vi "Create From Elements.vi"(7 "Mutable (F)":bool, 8 "error in (no error)":errorcluster, 10 "Elements":T1[](array[typedef])) -> (0 "error out":errorcluster, 3 "Config Manager out":refnum<class "Config Manager.lvclass">)   [LabVIEW 2023, in "CDM-Config.lvlib" / "Config Manager.lvclass"]
uses:
  Config Manager.lvclass
  Config Element.ctl
  Meta Data.ctl
  Value Type.ctl
  Config Element/Element Data.ctl
  Node Info.ctl
  Config Manager.lvclass/Config Manager.ctl
  CDM-Config.lvlib
  Config Element/Config Element.lvclass
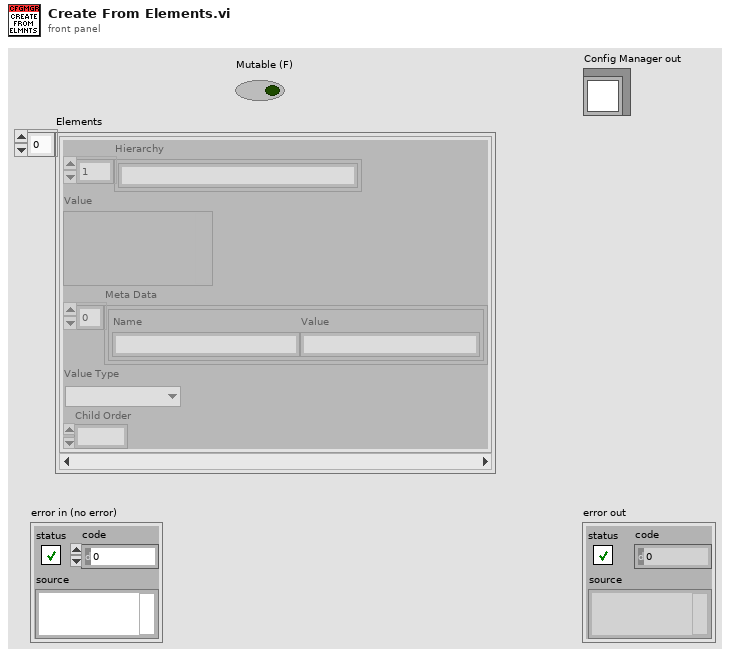
[diagram p1: front panel]
types:
  T1 = typedef "CDM-Config.lvlib/Config Element.ctl" = cluster{"Hierarchy":string[], "Value":variant, "Meta Data":T2[], "Value Type":T3, "Child Order":i32}
  T2 = typedef "CDM-Config.lvlib/Meta Data.ctl" = cluster{"Name":string, "Value":string}
  T3 = typedef "CDM-Config.lvlib/Value Type.ctl" = enum16{"String", "Number", "Bool", "Object", "Array"}
  T4 = typedef "CDM-Config.lvlib/Config Element.lvclass/Element Data.ctl" = cluster{"Node Info":T5, "Owner":refnum<class>, "Changed":bool, "Name":string, "Meta Data":T2[], "Value Type":T3, "Value":variant}
  T5 = typedef "CDM-Config.lvlib/Node Info.ctl" = cluster{"Index":i32, "Parent":i32, "Children":i32[]}
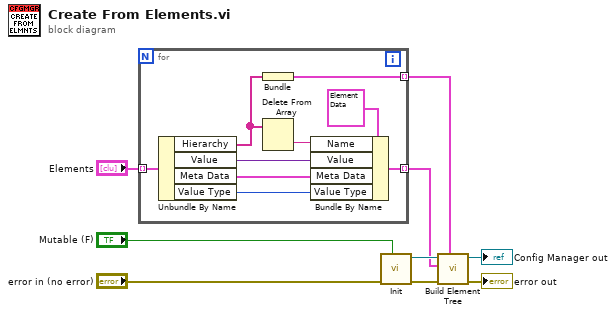
[diagram p0: block diagram]
diagram:
  n1 = for {
    tunnel: "Elements" -> [w18] mode=indexing
    tunnel: [w10] -> w4 mode=indexing
    tunnel: [w16] -> w3 mode=indexing
    n2 = Unbundle By Name(w18) -> ("Hierarchy"=w17:string[], "Value"=w13:variant, "Meta Data"=w12:T2[], "Value Type"=w11:T3)
    n3 = Bundle("Hierarchy"=w17) -> (w16:cluster{"Hierarchy":string[]})  [unwired: 1 in]
    n4 = Delete From Array(array=w17) -> (deleted portion=w14:string)  [unwired: 2 in, 1 out]
    n5 = Bundle By Name(cluster=T4 {"Node Info"={"Index"=-1, "Parent"=-1, "Children"=[]}, "Owner"=refnum, "Changed"=FALSE, "Name"="", "Meta Data"=[], "Value Type"=enum."String", "Value"=variant} ("Ref Data"), "Name"=w14, "Value"=w13, "Meta Data"=w12, "Value Type"=w11) -> (w10:T4)
  }
  n6 = call "Init.vi"("Mutable (F)"="Mutable (F)", "error in (no error)"="error in (no error)") -> ("error out"=w2:errorcluster, "Config Manager out"=w9:refnum<class "Config Manager.lvclass">)  [unwired: 8 in]
  n7 = call "Build Element Tree.vi"("Hierarchies"=w3, "error in (no error)"=w2, "Elements in"=w4, "Config Manager in"=w9) -> ("error out"=→"error out":errorcluster, "Config Manager out"=→"Config Manager out":refnum<class "Config Manager.lvclass">)  [unwired: 6 in]
